vi "roboRIO v1.0 Create Configuration List.vi"() -> (3 "Bitmask Array":bool[][](array[boolean]))   [LabVIEW 2021]
panel:
  # "This VI is provided for convenience so that the creation of the bitmask array used for configuring the functions is done in a single place. Therefore, any changes can be made here instead of in every single Build MUX Configuration XXX VI."
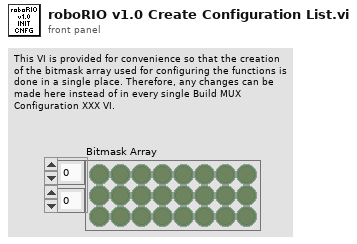
[diagram p1: front panel]
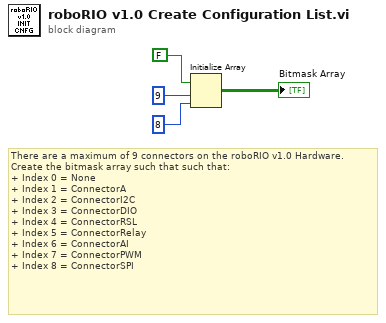
[diagram p0: block diagram]
diagram:
  # "There are a maximum of 9 connectors on the roboRIO v1.0 Hardware.\nCreate the bitmask array such that such that:\n+ Index 0 = None\n+ Index 1 = ConnectorA\n+ Index 2 = ConnectorI2C \n+ Index 3 = ConnectorDIO\n+ Index 4 = ConnectorRSL\n+ Index 5 = ConnectorRelay\n+ Index 6 = ConnectorAI\n+ Index 7 = ConnectorPWM\n+ Index 8 = ConnectorSPI"
  n1 = Initialize Array(FALSE, 9 ("dimension size"), 8 ("dimension size")) -> (→"Bitmask Array":bool[][])
